vi "CMD Start TDMS Logging.vi"(8 "error in (no error)":errorcluster, 11 "LogEngine in":refnum<class "LogEngine.lvclass">) -> (0 "error out":errorcluster, 3 "LogEngine out":refnum<class "LogEngine.lvclass">)   [LabVIEW 2017, in "LogEngine.lvclass"]
doc: "Developed by Kevin Thompson\nkevin@thompsonengineering.net\n\nCopyright 2018-2020\nThompson Engineering, LLC"
uses:
  LogEngine.lvclass
  Data Types/AsyncCmd_LogEngine--enum.ctl
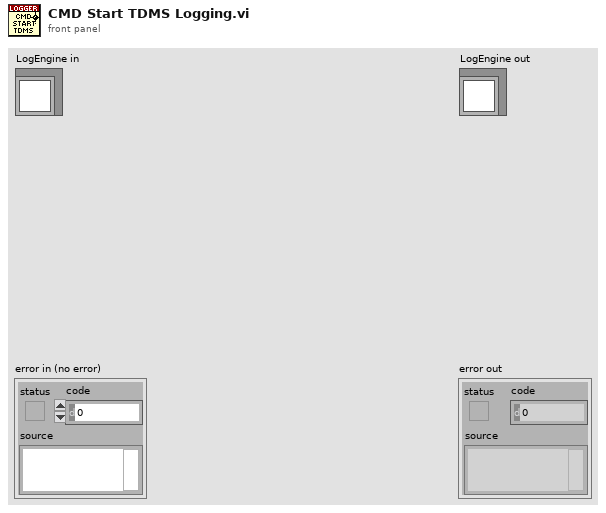
[diagram p1: front panel]
types:
  T1 = typedef "LogEngine.lvclass/AsyncCmd_LogEngine--enum.ctl" = enum16{"LE.CreateLogFile", "LE.EnableLogging", "LE.OpenTDMS", "LE.CloseTDMS", "LE.StartTDMSLogging", "LE.StopTDMSLogging"}
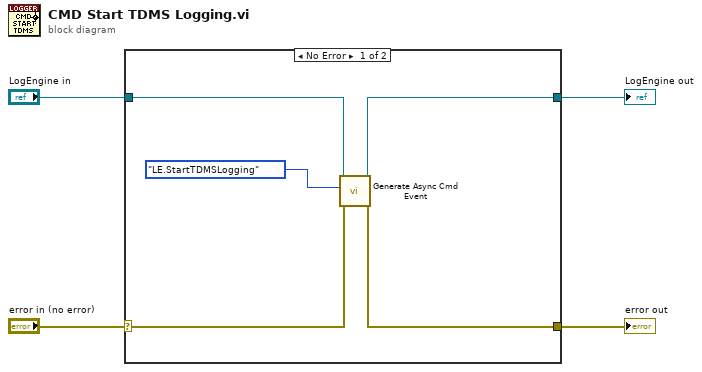
[diagram p0: block diagram]
diagram:
  n1 = case shown="No Error" "error in (no error)" {
    selector: "error in (no error)" -> [w9 w11]
    tunnel: [w8 w11] -> w3
    tunnel: [w7 w10] -> w1
    tunnel: "LogEngine in" -> [w6 w10]
    frame No Error {
      n2 = call "Generate Async Cmd Event.vi"("error in (no error)"=w9, "AsyncCmd"=AsyncCmd_LogEngine--enum."LE.StartTDMSLogging", "LogEngine"=w6) -> ("error out"=w8:errorcluster, "LogEngine out"=w7:refnum<class "LogEngine.lvclass">)  [unwired: 7 in]
    }
    frame Error {
    }
  }
  "error out" <- w3
  "LogEngine out" <- w1
